vi "MW_Display_Py_Get_Signal_Status.vi"(0 "session in":refnum<k35>, 5 "module path":path=path "D:/dev/Guy_Storage/Work/Cancun/MW_Display_Test/Magewell Capture/Capture_LV.py", 11 "error in":errorcluster) -> (4 "session out":refnum<k35>, 6 "module path out":path, 14 "Signal Status":T1, 15 "error out":errorcluster)   [LabVIEW 2023]
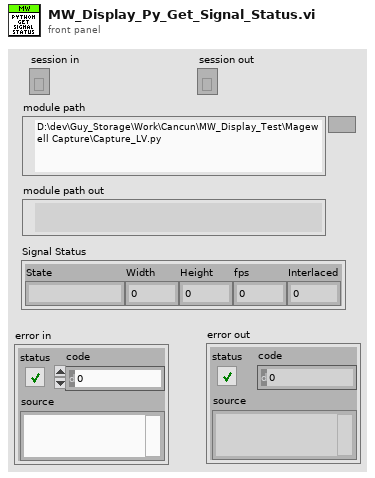
[diagram p1: front panel]
types:
  T1 = cluster{"State":string, "Width":i32, "Height":i32, "fps":i32, "Interlaced":i32}
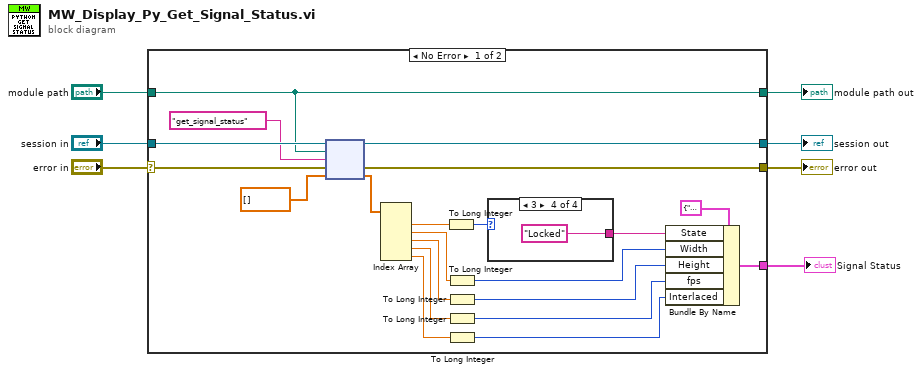
[diagram p0: block diagram]
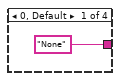
[diagram p2: hidden frame]
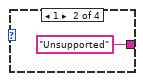
[diagram p3: hidden frame]
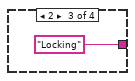
[diagram p4: hidden frame]
diagram:
  n1 = case shown="No Error" "error in" {
    selector: "error in" -> [w25 w34]
    tunnel: "module path" -> [w23 w33]
    tunnel: "session in" -> [w28 w35]
    tunnel: [w27 w34] -> w3
    tunnel: [w26 w35] -> w5
    tunnel: [w23 w33] -> w2
    tunnel: [w10 _] -> w1
    frame No Error {
      n2 = node(w28, w23, "get_signal_status" ("function name"), w25, dbl[] []) -> (w26:refnum<k35>, w27:errorcluster, w21:dbl[])  [unwired: 2 out]
      n3 = Index Array(array=w21) -> (element #1=w20:dbl, element #2=w18:dbl, element #3=w17:dbl, element #4=w16:dbl, element #5=w9:dbl)  [unwired: 5 in]
      n4 = To Long Integer(number=w20) -> (32bit integer=w19:i32)
      n5 = To Long Integer(number=w18) -> (32bit integer=w13:i32)
      n6 = To Long Integer(number=w17) -> (32bit integer=w12:i32)
      n7 = To Long Integer(number=w16) -> (32bit integer=w11:i32)
      n8 = To Long Integer(number=w9) -> (32bit integer=w8:i32)
      n9 = case shown="3" w19 {
        tunnel: ["None" "Unsupported" "Locking" "Locked"] -> w15
        frame 0, Default {
        }
        frame 1 {
        }
        frame 2 {
        }
        frame 3 {
        }
      }
      n10 = Bundle By Name(cluster=T1 {"State"="Locked", "Width"=0, "Height"=0, "fps"=0, "Interlaced"=0}, "State"=w15, "Width"=w13, "Height"=w12, "fps"=w11, "Interlaced"=w8) -> (w10:T1)
    }
    frame Error {
    }
  }
  "session out" <- w5
  "error out" <- w3
  "module path out" <- w2
  "Signal Status" <- w1
